vi "测试类型1自动测试一组 - 副本.vi"(7 "选择？":bool, 9 "第几个":i32) -> ()   [LabVIEW 2010]
uses:
  全局量/试验配置信息.vi
  全局量/自动测试结果.vi
panel:
  in  "测试值":dbl[](array[numeric])
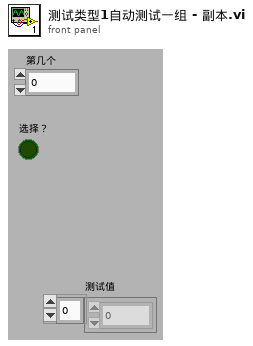
[diagram p1: front panel]
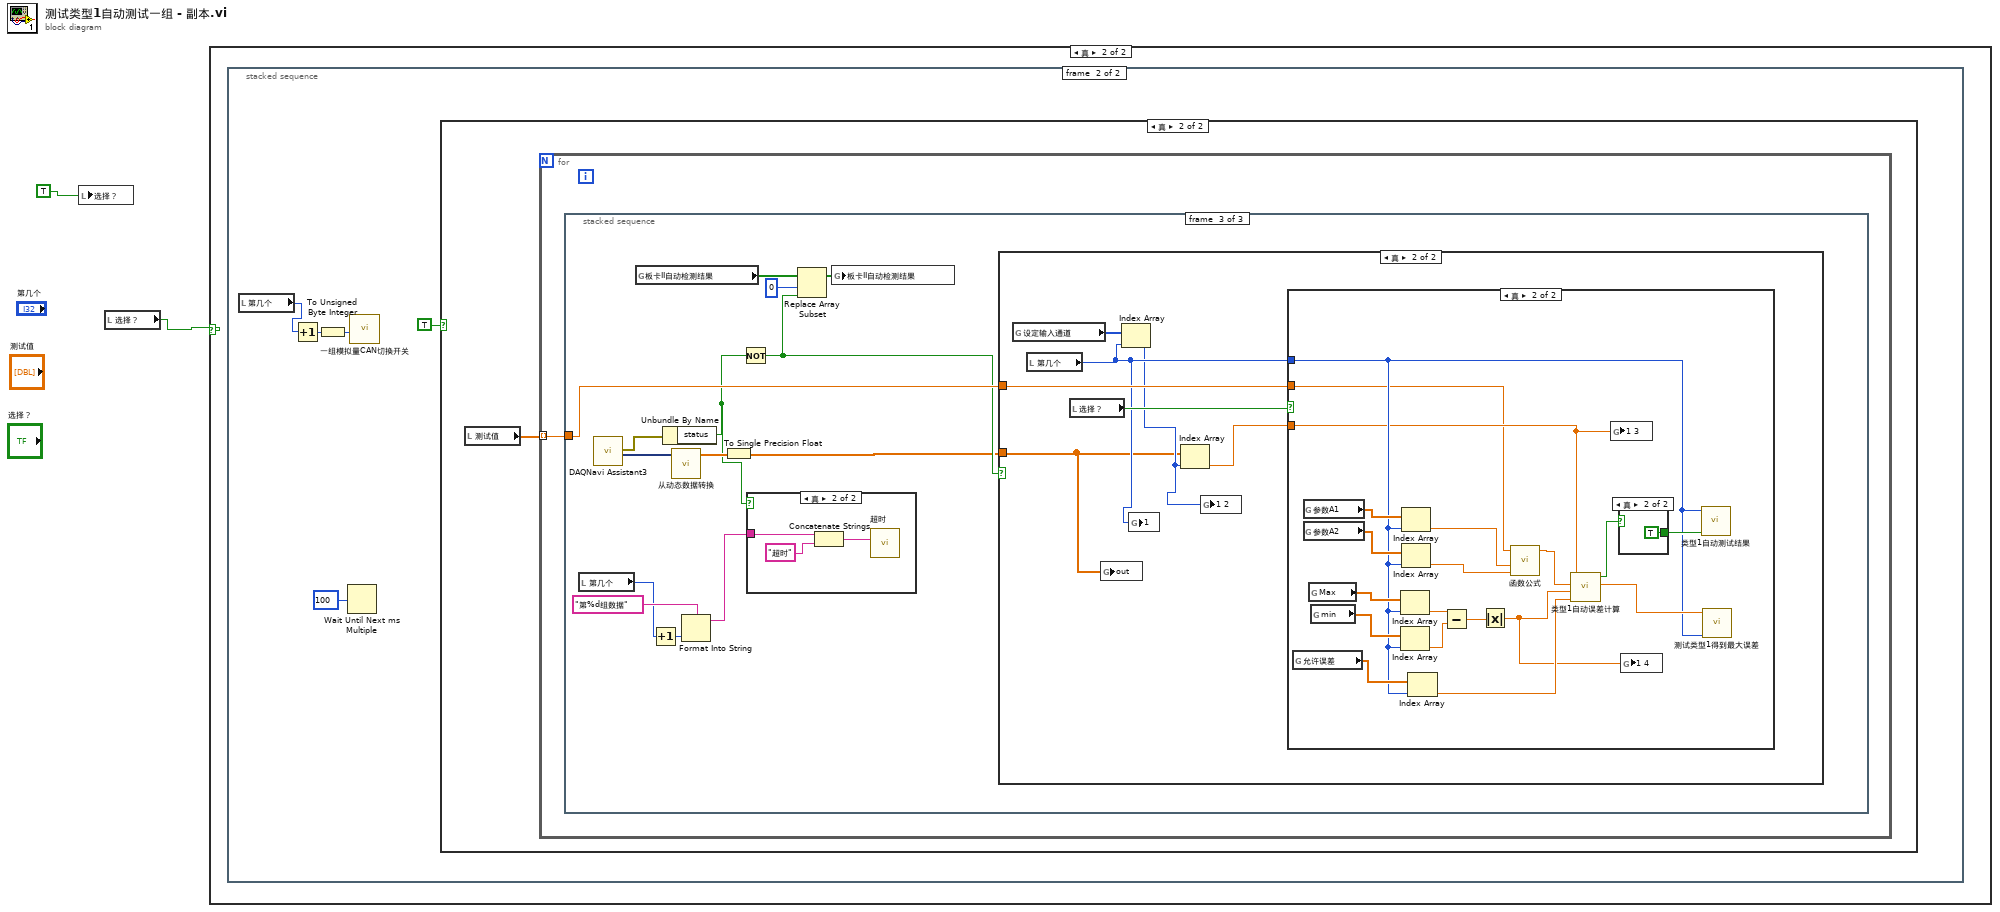
[diagram p0: block diagram]
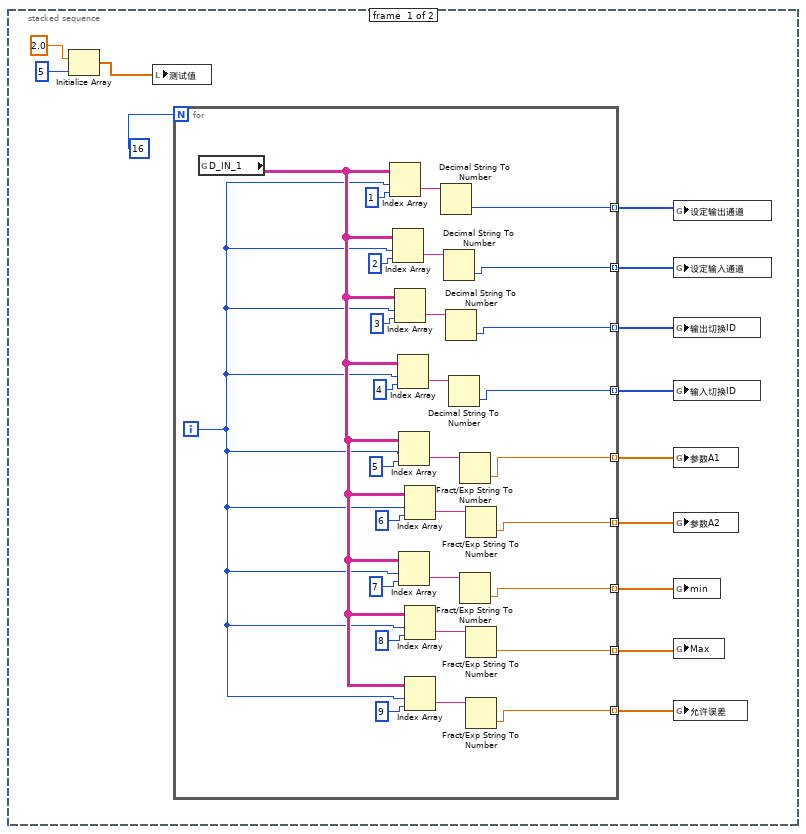
[diagram p3: hidden frame]
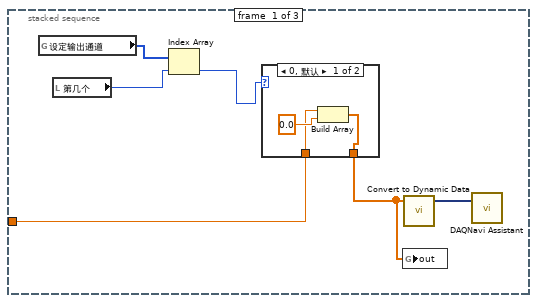
[diagram p5: hidden frame]
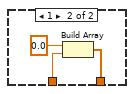
[diagram p6: hidden frame]
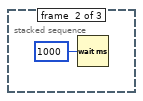
[diagram p7: hidden frame]
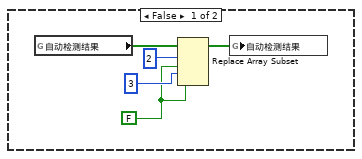
[diagram p9: hidden frame]
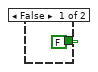
[diagram p11: hidden frame]
diagram:
  n1 = local write "选择？"(TRUE) -> ()
  n2 = local read "选择？"() -> (w2:bool)
  n3 = case shown="真" w2 {
    frame False {
    }
    frame True {
      n4 = stacked-sequence {
        frame #0 {
          n5 = Initialize Array(2.0, 5 ("维数大小")) -> (w15:dbl[])
          n6 = local write "测试值"(w15) -> ()
          n7 = for {
            N: 16 ("维数大小") -> [_]
            tunnel: [w24] -> w11 mode=indexing
            tunnel: [w23] -> w10 mode=indexing
            tunnel: [w22] -> w9 mode=indexing
            tunnel: [w21] -> w8 mode=indexing
            tunnel: [w20] -> w7 mode=indexing
            tunnel: [w19] -> w6 mode=indexing
            tunnel: [w18] -> w5 mode=indexing
            tunnel: [w17] -> w4 mode=indexing
            tunnel: [w16] -> w3 mode=indexing
            i -> [w25]
            n8 = global read "试验配置信息.vi" "D_IN_1"() -> (w26:string[][])
            n9 = Index Array(array=w26, index (row)=w25, index (col)=1 ("禁用的索引 (列)")) -> (element=w44:string)
            n10 = Index Array(array=w26, index (row)=w25, index (col)=2 ("禁用的索引 (列)")) -> (element=w41:string)
            n11 = Index Array(array=w26, index (row)=w25, index (col)=3 ("禁用的索引 (列)")) -> (element=w37:string)
            n12 = Index Array(array=w26, index (row)=w25, index (col)=4 ("禁用的索引 (列)")) -> (element=w40:string)
            n13 = Index Array(array=w26, index (row)=w25, index (col)=5 ("禁用的索引 (列)")) -> (element=w35:string)
            n14 = Index Array(array=w26, index (row)=w25, index (col)=7 ("禁用的索引 (列)")) -> (element=w30:string)
            n15 = Index Array(array=w26, index (row)=w25, index (col)=6 ("禁用的索引 (列)")) -> (element=w34:string)
            n16 = Index Array(array=w26, index (row)=w25, index (col)=8 ("禁用的索引 (列)")) -> (element=w31:string)
            n17 = Index Array(array=w26, index (row)=w25, index (col)=9 ("禁用的索引 (列)")) -> (element=w28:string)
            n18 = Decimal String To Number(string=w44) -> (number=w24:i32)  [unwired: 2 in, 1 out]
            n19 = Decimal String To Number(string=w41) -> (number=w23:i32)  [unwired: 2 in, 1 out]
            n20 = Decimal String To Number(string=w37) -> (number=w22:i32)  [unwired: 2 in, 1 out]
            n21 = Decimal String To Number(string=w40) -> (number=w21:i32)  [unwired: 2 in, 1 out]
            n22 = Fract/Exp String To Number(string=w35) -> (number=w20:dbl)  [unwired: 3 in, 1 out]
            n23 = Fract/Exp String To Number(string=w30) -> (number=w18:dbl)  [unwired: 3 in, 1 out]
            n24 = Fract/Exp String To Number(string=w34) -> (number=w19:dbl)  [unwired: 3 in, 1 out]
            n25 = Fract/Exp String To Number(string=w31) -> (number=w17:dbl)  [unwired: 3 in, 1 out]
            n26 = Fract/Exp String To Number(string=w28) -> (number=w16:dbl)  [unwired: 3 in, 1 out]
          }
          n27 = global write "试验配置信息.vi" "设定输出通道"(w11) -> ()
          n28 = global write "试验配置信息.vi" "设定输入通道"(w10) -> ()
          n29 = global write "试验配置信息.vi" "输出切换ID"(w9) -> ()
          n30 = global write "试验配置信息.vi" "输入切换ID"(w8) -> ()
          n31 = global write "试验配置信息.vi" "参数A1"(w7) -> ()
          n32 = global write "试验配置信息.vi" "参数A2"(w6) -> ()
          n33 = global write "试验配置信息.vi" "min"(w5) -> ()
          n34 = global write "试验配置信息.vi" "Max"(w4) -> ()
          n35 = global write "试验配置信息.vi" "允许误差"(w3) -> ()
        }
        frame #1 {
          n36 = local read "第几个"() -> (w46:i32)
          n37 = Increment(x=w46) -> (x+1=w48:i32)
          n38 = To Unsigned Byte Integer(number=w48) -> (unsigned 8bit integer=w49:u8)
          n39 = Wait Until Next ms Multiple(millisecond multiple=u32 100 ("毫秒倍数")) -> ()  [unwired: 1 out]
          n40 = call "一组模拟量CAN切换开关.vi"("第几组数据"=w49) -> ()  [unwired: 10 in, 1 out]
          n41 = case shown="真" TRUE {
            frame False {
            }
            frame True {
              n42 = local read "测试值"() -> (w50:dbl[])
              n43 = for {
                tunnel: w50 -> [w51] mode=indexing
                n44 = stacked-sequence {
                  tunnel: w51 -> [w54 _ w78]
                  frame #0 {
                    n45 = global read "试验配置信息.vi" "设定输出通道"() -> (w56:i32[])
                    n46 = local read "第几个"() -> (w55:i32)
                    n47 = Index Array(array=w56, index=w55) -> (element=w53:i32)
                    n48 = case shown="0, 默认" w53 {
                      tunnel: [w60 w63] -> w52
                      tunnel: w54 -> [w58 w61]
                      frame 0, Default {
                        n49 = Build Array(w58, 0.0) -> (w60:dbl[])
                      }
                      frame 1 {
                        n50 = Build Array(0.0, w61) -> (w63:dbl[])
                      }
                    }
                    n51 = global write "自动测试结果.vi" "out"(w52) -> ()
                    n52 = call "Convert to Dynamic Data"("Array"=w52) -> ("Dynamic Data Type"=w57:dynamicdata)  [unwired: 3 out]
                    n53 = call "DAQNavi Assistant"("data in(DDT)"=w57) -> ()  [unwired: 2 in, 17 out]
                  }
                  frame #1 {
                    n54 = Wait (ms)(milliseconds to wait=u32 1000 ("等待时间（毫秒）")) -> ()  [unwired: 1 out]
                  }
                  frame #2 {
                    n55 = local read "第几个"() -> (w74:i32)
                    n56 = call "DAQNavi Assistant3"() -> ("error out"=w69:errorcluster, "data out(DDT)"=w68:dynamicdata)  [unwired: 2 in, 16 out]
                    n57 = global read "试验配置信息.vi" "板卡II自动检测结果"() -> (w71:bool[])
                    n58 = Increment(x=w74) -> (x+1=w75:i32)
                    n59 = Unbundle By Name(w69) -> ("status"=w65:bool)
                    n60 = call "从动态数据转换"("Dynamic Data Type"=w68) -> ("Array"=w67:dbl[])  [unwired: 3 in]
                    n61 = Format Into String(format string="第%d组数据" ("格式字符串"), w75) -> (resulting string=w76:string)  [unwired: 2 in, 1 out]
                    n62 = To Single Precision Float(number=w67) -> (single precision float=w66:sgl[])
                    n63 = Not(x=w65) -> (.not. x?=w70:bool)
                    n64 = case shown="真" w65 {
                      tunnel: w76 -> [_ w81]
                      frame False {
                      }
                      frame True {
                        n65 = Concatenate Strings(w81, "超时" ("格式字符串")) -> (w79:string)
                        n66 = call "超时"("Message"=w79) -> ()  [unwired: 9 in, 2 out]
                      }
                    }
                    n67 = Replace Array Subset(array=w71, new element=w70, index=0 ("索引")) -> (w72:bool[])
                    n68 = global write "试验配置信息.vi" "板卡II自动检测结果"(w72) -> ()
                    n69 = case shown="真" w70 {
                      tunnel: w78 -> [_ w92]
                      tunnel: w66 -> [_ w87]
                      frame False {
                        w82 = FALSE
                        n70 = global read "试验配置信息.vi" "自动检测结果"() -> (w85:bool[])
                        n71 = Replace Array Subset(array=w85, new element #1=w82, index #1=2 ("索引"), new element #2=w82, index #2=3 ("索引")) -> (w84:bool[])
                        n72 = global write "试验配置信息.vi" "自动检测结果"(w84) -> ()
                      }
                      frame True {
                        n73 = global read "试验配置信息.vi" "设定输入通道"() -> (w91:i32[])
                        n74 = local read "第几个"() -> (w89:i32)
                        n75 = local read "选择？"() -> (w93:bool)
                        n76 = global write "自动测试结果.vi" "out"(w87) -> ()
                        n77 = Index Array(array=w91, index=w89) -> (element=w88:i32)
                        n78 = global write "自动测试结果.vi" "1"(w89) -> ()
                        n79 = Index Array(array=w87, index=w88) -> (element=w90:sgl)
                        n80 = global write "自动测试结果.vi" "1 2"(w88) -> ()
                        n81 = case shown="真" w93 {
                          tunnel: w92 -> [_ w95]
                          tunnel: w90 -> [_ w98]
                          tunnel: w89 -> [_ w99]
                          frame False {
                          }
                          frame True {
                            n82 = global read "试验配置信息.vi" "允许误差"() -> (w108:dbl[])
                            n83 = global read "试验配置信息.vi" "参数A1"() -> (w112:dbl[])
                            n84 = global read "试验配置信息.vi" "参数A2"() -> (w111:dbl[])
                            n85 = global read "试验配置信息.vi" "Max"() -> (w109:dbl[])
                            n86 = global read "试验配置信息.vi" "min"() -> (w110:dbl[])
                            n87 = Index Array(array=w109, index=w99) -> (element=w106:dbl)
                            n88 = Index Array(array=w110, index=w99) -> (element=w105:dbl)
                            n89 = Index Array(array=w112, index=w99) -> (element=w96:dbl)
                            n90 = Index Array(array=w111, index=w99) -> (element=w104:dbl)
                            n91 = Index Array(array=w108, index=w99) -> (element=w103:dbl)
                            n92 = Subtract(x=w106, y=w105) -> (x-y=w107:dbl)
                            n93 = Absolute Value(x=w107) -> (abs(x)=w94:dbl)
                            n94 = call "函数公式.vi"("参数 b"=w104, "参数 a"=w96, "设定值 1"=w95) -> ("y"=w97:dbl)  [unwired: 5 in, 1 out]
                            n95 = call "类型1自动误差计算.vi"("允许误差"=w103, "模拟量量程范围"=w94, "设定值_1"=w97, "反馈值_1"=w98) -> ("误差_1"=w100:dbl, "合格_1?"=w102:bool)  [unwired: 5 in, 1 out]
                            n96 = global write "自动测试结果.vi" "1 3"(w98) -> ()
                            n97 = case shown="真" w102 {
                              tunnel: [FALSE TRUE] -> w101
                              frame False {
                              }
                              frame True {
                              }
                            }
                            n98 = global write "自动测试结果.vi" "1 4"(w94) -> ()
                            n99 = call "类型1自动测试结果.vi"("合格?"=w101, "第几个"=w99) -> ()  [unwired: 10 in]
                            n100 = call "测试类型1得到最大误差.vi"("第几组"=w99, "新误差值"=w100) -> ()  [unwired: 10 in]
                          }
                        }
                      }
                    }
                  }
                }
              }
            }
          }
        }
      }
    }
  }
